vi "write_parameteres_to_file.vi"(0 "error 2":errorcluster, 8 "error":errorcluster, 11 "vi path":path) -> ()   [LabVIEW 2019]
panel:
  in  "data values 3":variant[](array[variant])
  in  "data values 2":variant[](array[variant])
  out "save path":string
  in  "data values":variant[](array[variant])
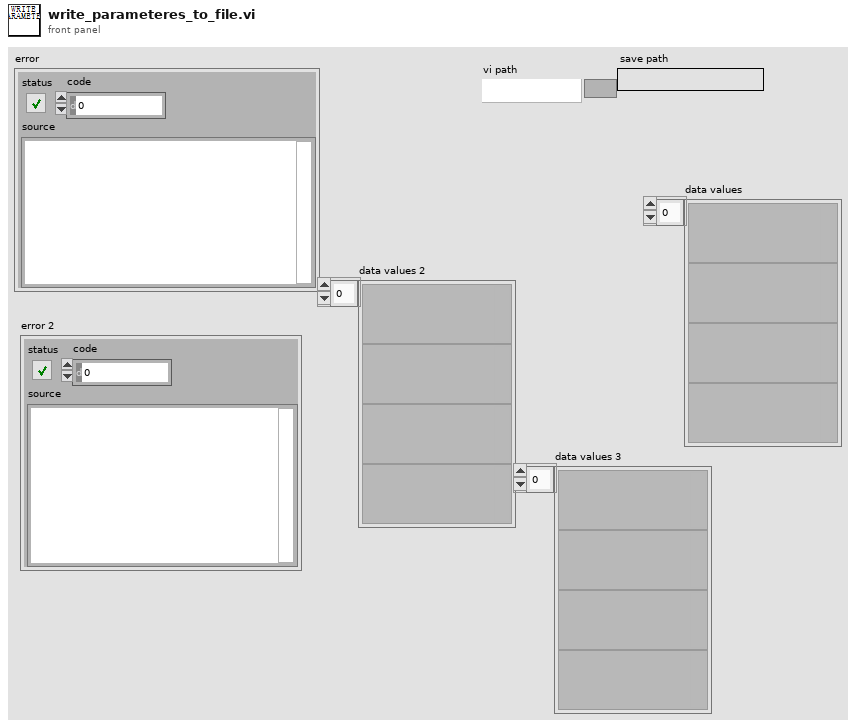
[diagram p1: front panel]
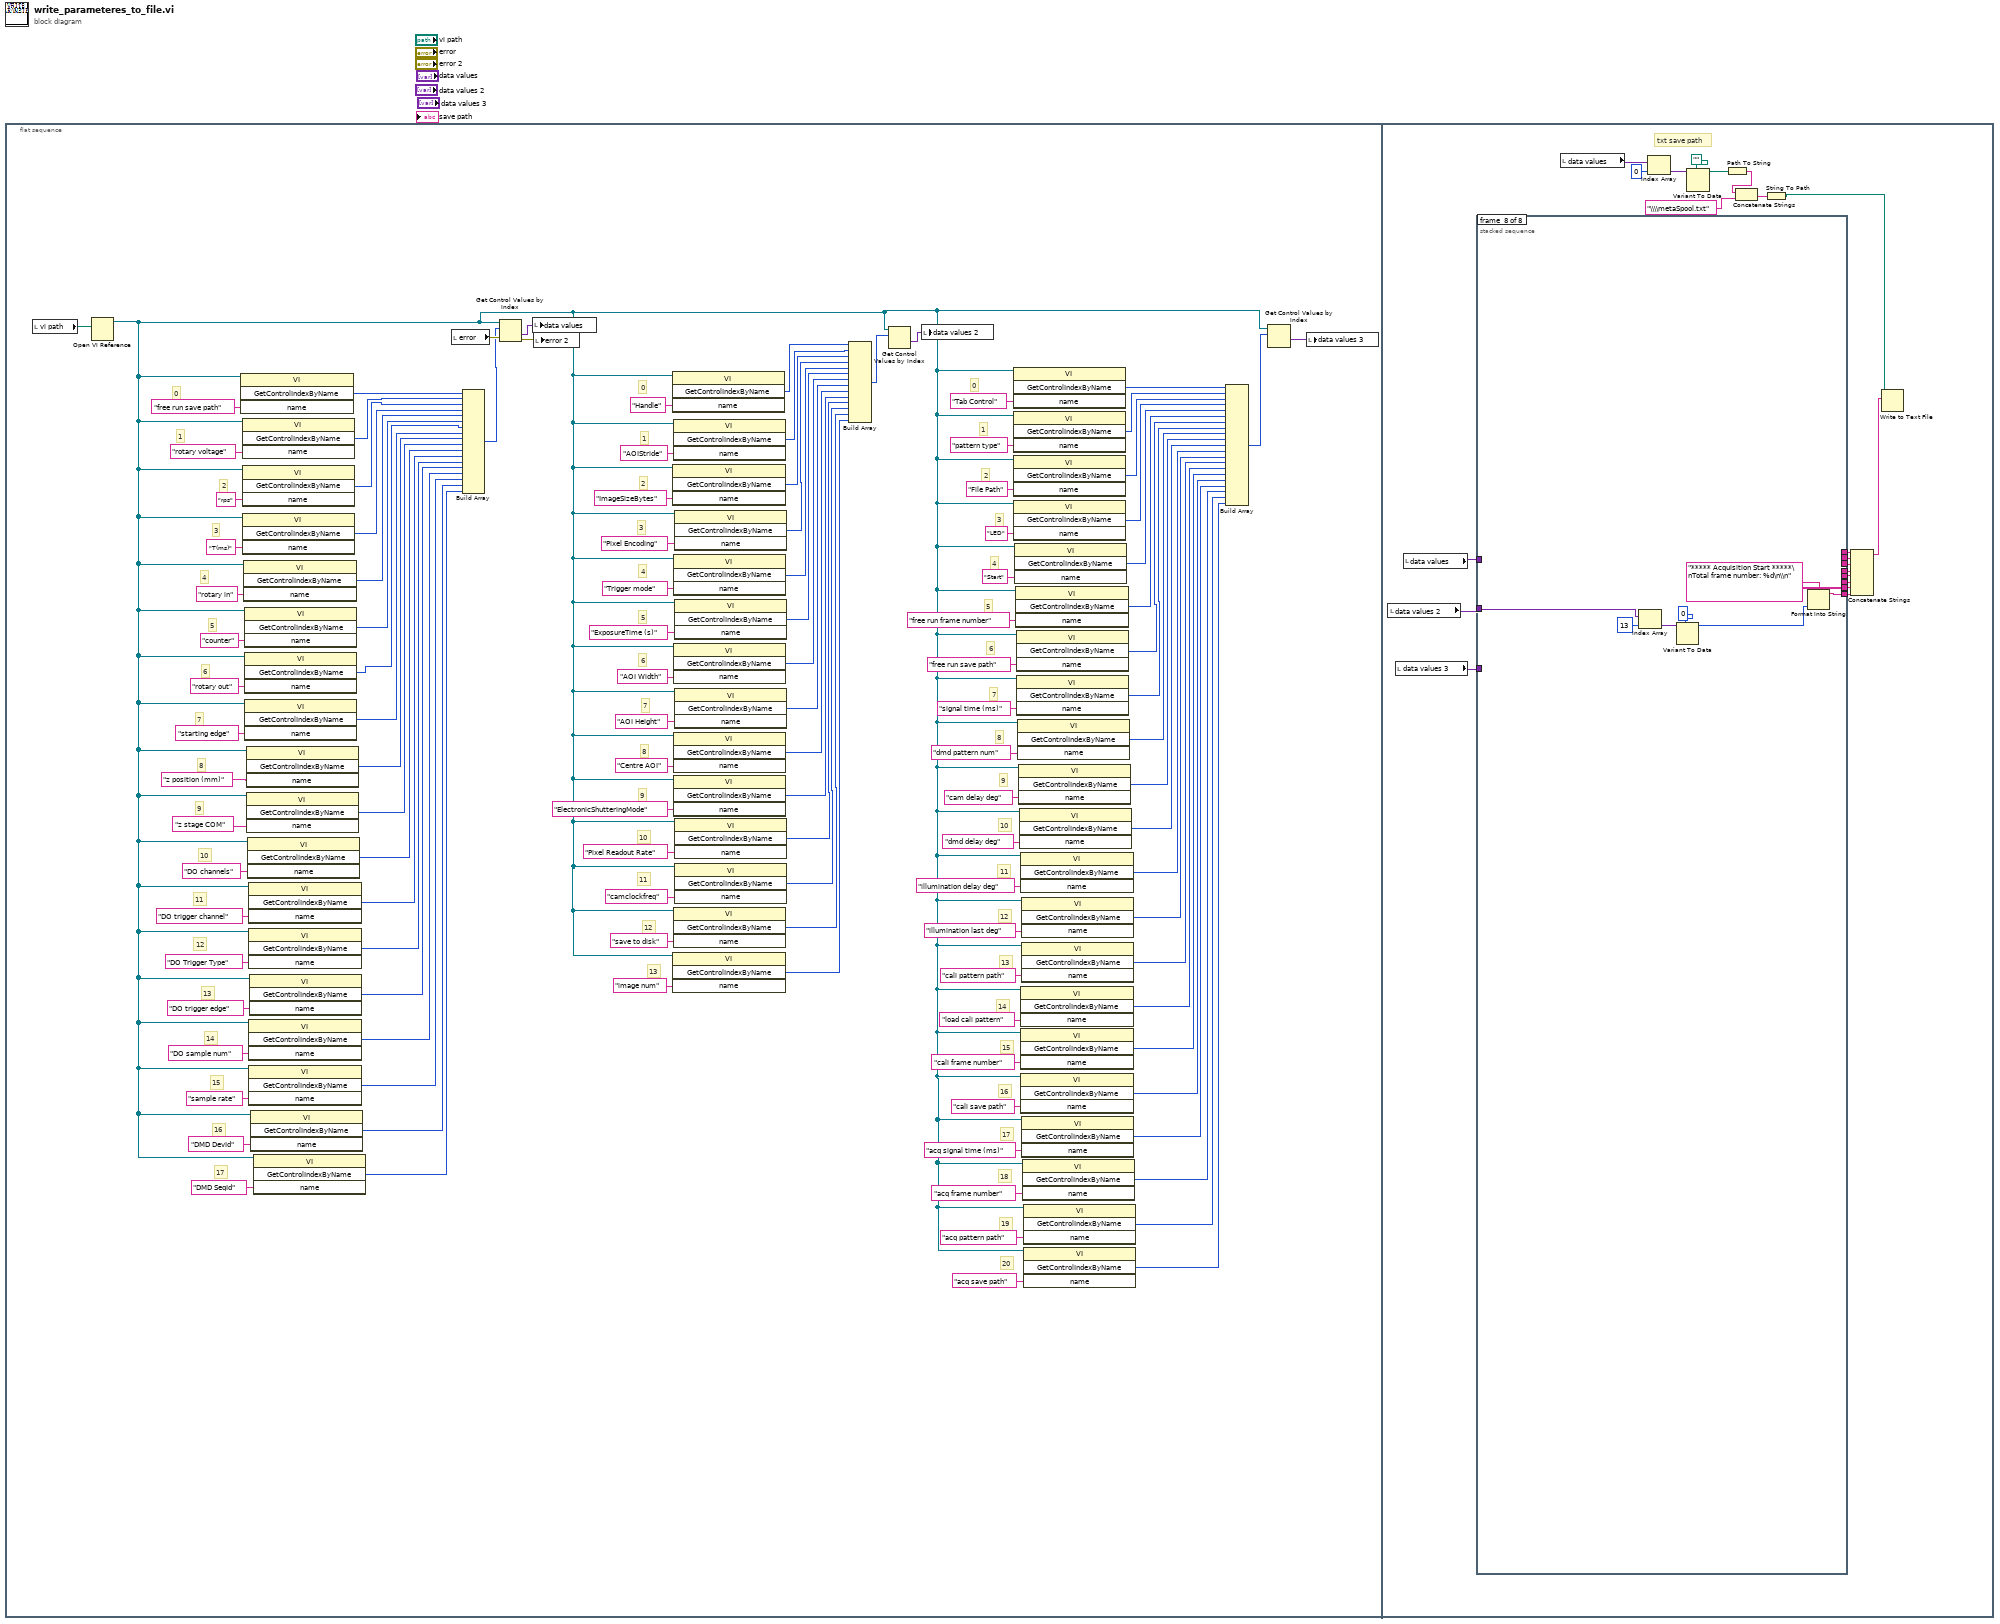
[diagram p0: block diagram]
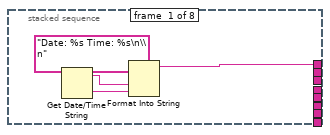
[diagram p2: hidden frame]
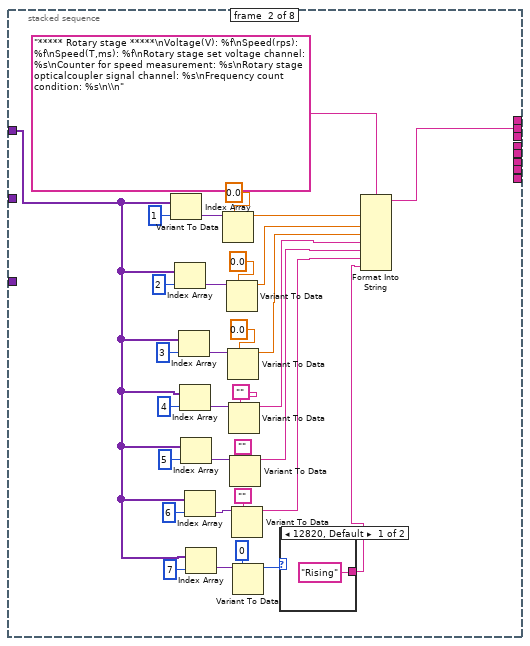
[diagram p3: hidden frame]
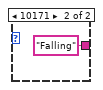
[diagram p4: hidden frame]
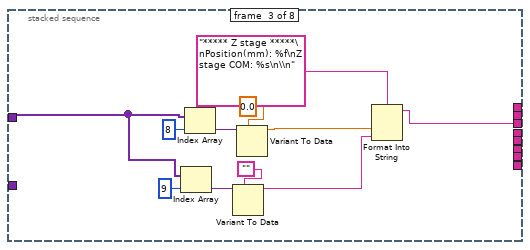
[diagram p5: hidden frame]
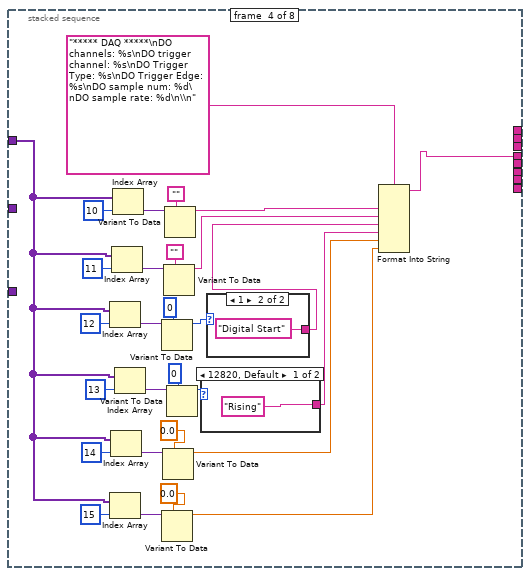
[diagram p6: hidden frame]
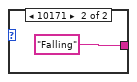
[diagram p7: hidden frame]
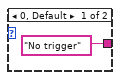
[diagram p8: hidden frame]
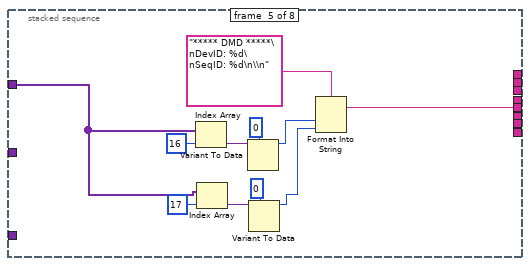
[diagram p9: hidden frame]
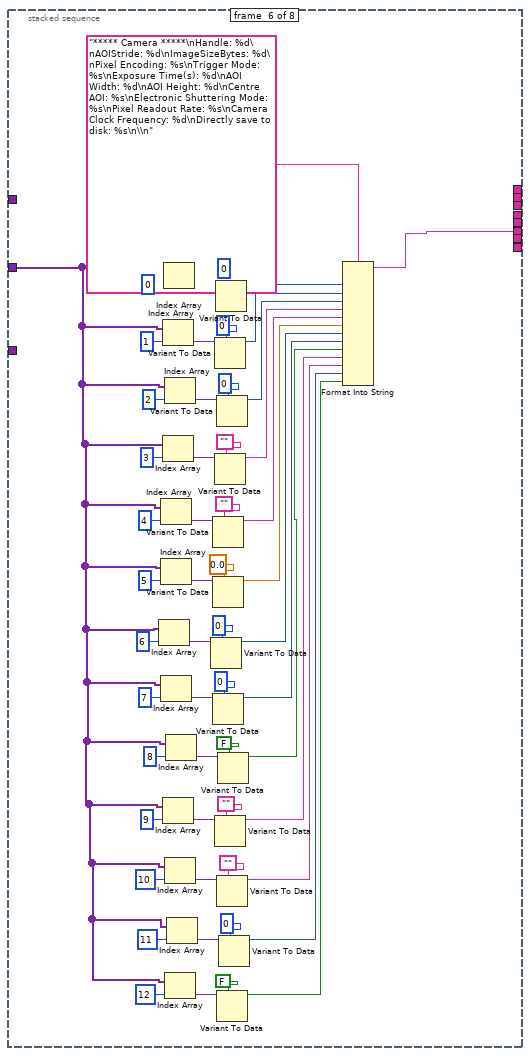
[diagram p10: hidden frame]
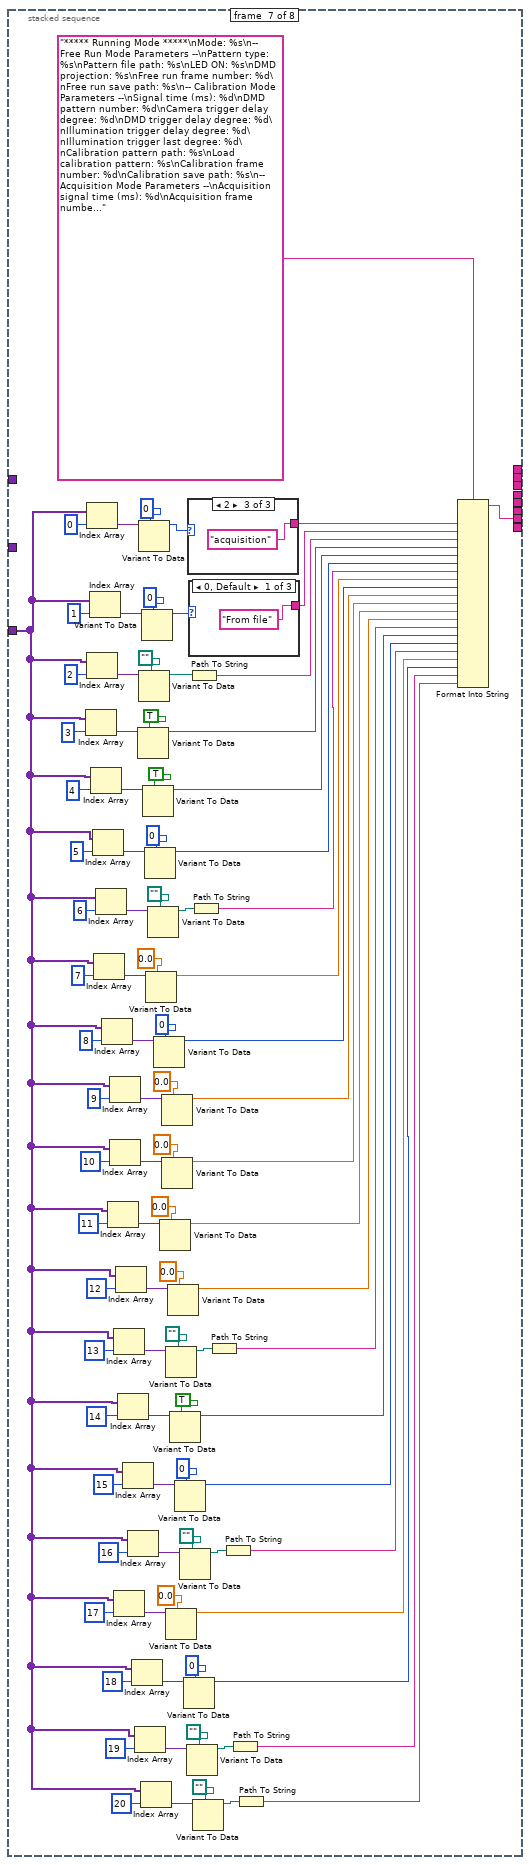
[diagram p11: hidden frame]
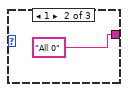
[diagram p12: hidden frame]
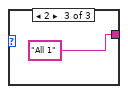
[diagram p13: hidden frame]
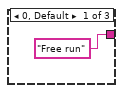
[diagram p14: hidden frame]
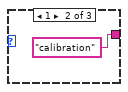
[diagram p15: hidden frame]
diagram:
  n1 = flat-sequence {
    frame #0 {
      # "13"
      # "15"
      # "20"
      # "19"
      # "18"
      # "17"
      # "16"
      # "14"
      # "13"
      # "12"
      # "11"
      # "10"
      # "9"
      # "8"
      # "7"
      # "6"
      # "5"
      # "4"
      # "3"
      # "2"
      # "1"
      # "12"
      # "0"
      # "11"
      # "10"
      # "9"
      # "8"
      # "7"
      # "6"
      # "5"
      # "4"
      # "3"
      # "2"
      # "1"
      # "0"
      # "17"
      # "16"
      # "15"
      # "14"
      # "13"
      # "12"
      # "11"
      # "10"
      # "9"
      # "8"
      # "7"
      # "6"
      # "5"
      # "4"
      # "3"
      # "2"
      # "1"
      # "0"
      n2 = local read "vi path"() -> (w116:path)
      n3 = Open VI Reference(vi path=w116) -> (vi reference=w2:refnum<vi>)  [unwired: 5 in, 1 out]
      n4 = invoke class="VI" method="GetControlIndexByName"(reference=w2, "name"="free run save path" ("Control Name")) -> ("GetControlIndexByName"=w108:i32)  [unwired: 2 in, 3 out]
      n5 = invoke class="VI" method="GetControlIndexByName"(reference=w2, "name"="rotary voltage" ("Control Name")) -> ("GetControlIndexByName"=w110:i32)  [unwired: 2 in, 3 out]
      n6 = invoke class="VI" method="GetControlIndexByName"(reference=w2, "name"="rps" ("Control Name")) -> ("GetControlIndexByName"=w105:i32)  [unwired: 2 in, 3 out]
      n7 = invoke class="VI" method="GetControlIndexByName"(reference=w2, "name"="T(ms)" ("Control Name")) -> ("GetControlIndexByName"=w104:i32)  [unwired: 2 in, 3 out]
      n8 = invoke class="VI" method="GetControlIndexByName"(reference=w2, "name"="rotary in" ("Control Name")) -> ("GetControlIndexByName"=w102:i32)  [unwired: 2 in, 3 out]
      n9 = invoke class="VI" method="GetControlIndexByName"(reference=w2, "name"="counter" ("Control Name")) -> ("GetControlIndexByName"=w100:i32)  [unwired: 2 in, 3 out]
      n10 = invoke class="VI" method="GetControlIndexByName"(reference=w2, "name"="rotary out" ("Control Name")) -> ("GetControlIndexByName"=w98:i32)  [unwired: 2 in, 3 out]
      n11 = invoke class="VI" method="GetControlIndexByName"(reference=w2, "name"="starting edge" ("Control Name")) -> ("GetControlIndexByName"=w97:i32)  [unwired: 2 in, 3 out]
      n12 = invoke class="VI" method="GetControlIndexByName"(reference=w2, "name"="z position (mm)" ("Control Name")) -> ("GetControlIndexByName"=w95:i32)  [unwired: 2 in, 3 out]
      n13 = invoke class="VI" method="GetControlIndexByName"(reference=w2, "name"="z stage COM" ("Control Name")) -> ("GetControlIndexByName"=w94:i32)  [unwired: 2 in, 3 out]
      n14 = invoke class="VI" method="GetControlIndexByName"(reference=w2, "name"="DO channels" ("Control Name")) -> ("GetControlIndexByName"=w83:i32)  [unwired: 2 in, 3 out]
      n15 = invoke class="VI" method="GetControlIndexByName"(reference=w2, "name"="DO trigger channel" ("Control Name")) -> ("GetControlIndexByName"=w82:i32)  [unwired: 2 in, 3 out]
      n16 = invoke class="VI" method="GetControlIndexByName"(reference=w2, "name"="DO Trigger Type" ("Control Name")) -> ("GetControlIndexByName"=w81:i32)  [unwired: 2 in, 3 out]
      n17 = invoke class="VI" method="GetControlIndexByName"(reference=w2, "name"="DO sample num" ("Control Name")) -> ("GetControlIndexByName"=w79:i32)  [unwired: 2 in, 3 out]
      n18 = invoke class="VI" method="GetControlIndexByName"(reference=w2, "name"="sample rate" ("Control Name")) -> ("GetControlIndexByName"=w78:i32)  [unwired: 2 in, 3 out]
      n19 = invoke class="VI" method="GetControlIndexByName"(reference=w2, "name"="DO trigger edge" ("Control Name")) -> ("GetControlIndexByName"=w80:i32)  [unwired: 2 in, 3 out]
      n20 = invoke class="VI" method="GetControlIndexByName"(reference=w2, "name"="DMD DevId" ("Control Name")) -> ("GetControlIndexByName"=w77:i32)  [unwired: 2 in, 3 out]
      n21 = invoke class="VI" method="GetControlIndexByName"(reference=w2, "name"="DMD SeqId" ("Control Name")) -> ("GetControlIndexByName"=w76:i32)  [unwired: 2 in, 3 out]
      n22 = local read "error"() -> (w115:errorcluster)
      n23 = Build Array(w108, w110, w105, w104, w102, w100, w98, w97, w95, w94, w83, w82, w81, w80, w79, w78, w77, w76) -> (w112:i32[])
      n24 = Get Control Values by Index(0:w2, 1:w112, 3:w115) -> (10:w109:variant[], 11:w114:errorcluster)
      n25 = local write "data values"(w109) -> ()
      n26 = local write "error 2"(w114) -> ()
      n27 = invoke class="VI" method="GetControlIndexByName"(reference=w2, "name"="Handle" ("Control Name")) -> ("GetControlIndexByName"=w73:i32)  [unwired: 2 in, 3 out]
      n28 = invoke class="VI" method="GetControlIndexByName"(reference=w2, "name"="ImageSizeBytes" ("Control Name")) -> ("GetControlIndexByName"=w59:i32)  [unwired: 2 in, 3 out]
      n29 = invoke class="VI" method="GetControlIndexByName"(reference=w2, "name"="image num" ("Control Name")) -> ("GetControlIndexByName"=w1:i32)  [unwired: 2 in, 3 out]
      n30 = invoke class="VI" method="GetControlIndexByName"(reference=w2, "name"="AOIStride" ("Control Name")) -> ("GetControlIndexByName"=w70:i32)  [unwired: 2 in, 3 out]
      n31 = invoke class="VI" method="GetControlIndexByName"(reference=w2, "name"="Trigger mode" ("Control Name")) -> ("GetControlIndexByName"=w57:i32)  [unwired: 2 in, 3 out]
      n32 = invoke class="VI" method="GetControlIndexByName"(reference=w2, "name"="AOI Width" ("Control Name")) -> ("GetControlIndexByName"=w55:i32)  [unwired: 2 in, 3 out]
      n33 = invoke class="VI" method="GetControlIndexByName"(reference=w2, "name"="Centre AOI" ("Control Name")) -> ("GetControlIndexByName"=w53:i32)  [unwired: 2 in, 3 out]
      n34 = invoke class="VI" method="GetControlIndexByName"(reference=w2, "name"="ElectronicShutteringMode" ("Control Name")) -> ("GetControlIndexByName"=w52:i32)  [unwired: 2 in, 3 out]
      n35 = invoke class="VI" method="GetControlIndexByName"(reference=w2, "name"="save to disk" ("Control Name")) -> ("GetControlIndexByName"=w38:i32)  [unwired: 2 in, 3 out]
      n36 = invoke class="VI" method="GetControlIndexByName"(reference=w2, "name"="Pixel Encoding" ("Control Name")) -> ("GetControlIndexByName"=w58:i32)  [unwired: 2 in, 3 out]
      n37 = invoke class="VI" method="GetControlIndexByName"(reference=w2, "name"="ExposureTime (s)" ("Control Name")) -> ("GetControlIndexByName"=w56:i32)  [unwired: 2 in, 3 out]
      n38 = invoke class="VI" method="GetControlIndexByName"(reference=w2, "name"="AOI Height" ("Control Name")) -> ("GetControlIndexByName"=w54:i32)  [unwired: 2 in, 3 out]
      n39 = invoke class="VI" method="GetControlIndexByName"(reference=w2, "name"="Pixel Readout Rate" ("Control Name")) -> ("GetControlIndexByName"=w51:i32)  [unwired: 2 in, 3 out]
      n40 = invoke class="VI" method="GetControlIndexByName"(reference=w2, "name"="camclockfreq" ("Control Name")) -> ("GetControlIndexByName"=w50:i32)  [unwired: 2 in, 3 out]
      n41 = Build Array(w73, w70, w59, w58, w57, w56, w55, w54, w53, w52, w51, w50, w38, w1) -> (w74:i32[])
      n42 = Get Control Values by Index(0:w2, 1:w74) -> (10:w75:variant[])  [unwired: 1 in, 1 out]
      n43 = local write "data values 2"(w75) -> ()
      n44 = invoke class="VI" method="GetControlIndexByName"(reference=w2, "name"="Tab Control" ("Control Name")) -> ("GetControlIndexByName"=w48:i32)  [unwired: 2 in, 3 out]
      n45 = invoke class="VI" method="GetControlIndexByName"(reference=w2, "name"="pattern type" ("Control Name")) -> ("GetControlIndexByName"=w33:i32)  [unwired: 2 in, 3 out]
      n46 = invoke class="VI" method="GetControlIndexByName"(reference=w2, "name"="File Path" ("Control Name")) -> ("GetControlIndexByName"=w32:i32)  [unwired: 2 in, 3 out]
      n47 = invoke class="VI" method="GetControlIndexByName"(reference=w2, "name"="LED" ("Control Name")) -> ("GetControlIndexByName"=w31:i32)  [unwired: 2 in, 3 out]
      n48 = invoke class="VI" method="GetControlIndexByName"(reference=w2, "name"="Start" ("Control Name")) -> ("GetControlIndexByName"=w30:i32)  [unwired: 2 in, 3 out]
      n49 = invoke class="VI" method="GetControlIndexByName"(reference=w2, "name"="free run frame number" ("Control Name")) -> ("GetControlIndexByName"=w29:i32)  [unwired: 2 in, 3 out]
      n50 = invoke class="VI" method="GetControlIndexByName"(reference=w2, "name"="free run save path" ("Control Name")) -> ("GetControlIndexByName"=w28:i32)  [unwired: 2 in, 3 out]
      n51 = invoke class="VI" method="GetControlIndexByName"(reference=w2, "name"="signal time (ms)" ("Control Name")) -> ("GetControlIndexByName"=w27:i32)  [unwired: 2 in, 3 out]
      n52 = invoke class="VI" method="GetControlIndexByName"(reference=w2, "name"="dmd pattern num" ("Control Name")) -> ("GetControlIndexByName"=w26:i32)  [unwired: 2 in, 3 out]
      n53 = invoke class="VI" method="GetControlIndexByName"(reference=w2, "name"="cam delay deg" ("Control Name")) -> ("GetControlIndexByName"=w25:i32)  [unwired: 2 in, 3 out]
      n54 = invoke class="VI" method="GetControlIndexByName"(reference=w2, "name"="dmd delay deg" ("Control Name")) -> ("GetControlIndexByName"=w24:i32)  [unwired: 2 in, 3 out]
      n55 = invoke class="VI" method="GetControlIndexByName"(reference=w2, "name"="illumination delay deg" ("Control Name")) -> ("GetControlIndexByName"=w18:i32)  [unwired: 2 in, 3 out]
      n56 = invoke class="VI" method="GetControlIndexByName"(reference=w2, "name"="load cali pattern" ("Control Name")) -> ("GetControlIndexByName"=w15:i32)  [unwired: 2 in, 3 out]
      n57 = invoke class="VI" method="GetControlIndexByName"(reference=w2, "name"="cali frame number" ("Control Name")) -> ("GetControlIndexByName"=w6:i32)  [unwired: 2 in, 3 out]
      n58 = invoke class="VI" method="GetControlIndexByName"(reference=w2, "name"="cali save path" ("Control Name")) -> ("GetControlIndexByName"=w5:i32)  [unwired: 2 in, 3 out]
      n59 = invoke class="VI" method="GetControlIndexByName"(reference=w2, "name"="illumination last deg" ("Control Name")) -> ("GetControlIndexByName"=w17:i32)  [unwired: 2 in, 3 out]
      n60 = invoke class="VI" method="GetControlIndexByName"(reference=w2, "name"="cali pattern path" ("Control Name")) -> ("GetControlIndexByName"=w16:i32)  [unwired: 2 in, 3 out]
      n61 = invoke class="VI" method="GetControlIndexByName"(reference=w2, "name"="acq signal time (ms)" ("Control Name")) -> ("GetControlIndexByName"=w4:i32)  [unwired: 2 in, 3 out]
      n62 = invoke class="VI" method="GetControlIndexByName"(reference=w2, "name"="acq frame number" ("Control Name")) -> ("GetControlIndexByName"=w7:i32)  [unwired: 2 in, 3 out]
      n63 = invoke class="VI" method="GetControlIndexByName"(reference=w2, "name"="acq pattern path" ("Control Name")) -> ("GetControlIndexByName"=w8:i32)  [unwired: 2 in, 3 out]
      n64 = invoke class="VI" method="GetControlIndexByName"(reference=w2, "name"="acq save path" ("Control Name")) -> ("GetControlIndexByName"=w9:i32)  [unwired: 2 in, 3 out]
      n65 = Build Array(w48, w33, w32, w31, w30, w29, w28, w27, w26, w25, w24, w18, w17, w16, w15, w6, w5, w4, w7, w8, w9) -> (w47:i32[])
      n66 = Get Control Values by Index(0:w2, 1:w47) -> (10:w49:variant[])  [unwired: 1 in, 1 out]
      n67 = local write "data values 3"(w49) -> ()
    }
    frame #1 {
      # "txt save path"
      n68 = local read "data values 2"() -> (w120:variant[])
      n69 = local read "data values 3"() -> (w118:variant[])
      n70 = local read "data values"() -> (w124:variant[])
      n71 = stacked-sequence {
        tunnel: [w138 _ _ _ _ _ _ _] -> w127
        tunnel: [_ w143 _ _ _ _ _ _] -> w126
        tunnel: [_ _ w177 _ _ _ _ _] -> w125
        tunnel: w124 -> [_ w142 w176 w188 w220 _ _ _]
        tunnel: [_ _ _ w204 _ _ _ _] -> w123
        tunnel: [_ _ _ _ w230 _ _ _] -> w122
        tunnel: [_ _ _ _ _ w281 _ _] -> w121
        tunnel: w120 -> [_ _ _ _ _ w232 _ w387]
        tunnel: [_ _ _ _ _ _ w377 _] -> w119
        tunnel: w118 -> [_ _ _ _ _ _ w296 _]
        tunnel: [_ _ _ _ _ _ _ w393] -> w117
        frame #0 {
          n72 = Get Date/Time String() -> (date string=w140:string, time string=w141:string)  [unwired: 3 in]
          n73 = Format Into String(format string="Date: %s Time: %s\n\\n", w140, w141) -> (resulting string=w138:string)  [unwired: 2 in, 1 out]
        }
        frame #1 {
          n74 = Index Array(array=w142, index=1) -> (element=w159:variant)
          n75 = Index Array(array=w142, index=2) -> (element=w161:variant)
          n76 = Index Array(array=w142, index=3) -> (element=w163:variant)
          n77 = Index Array(array=w142, index=4) -> (element=w165:variant)
          n78 = Index Array(array=w142, index=5) -> (element=w167:variant)
          n79 = Index Array(array=w142, index=6) -> (element=w169:variant)
          n80 = Index Array(array=w142, index=7) -> (element=w170:variant)
          n81 = Variant To Data(type=0.0, Variant=w159) -> (data=w160:dbl)  [unwired: 1 in, 1 out]
          n82 = Variant To Data(type=0.0, Variant=w161) -> (data=w162:dbl)  [unwired: 1 in, 1 out]
          n83 = Variant To Data(type=0.0, Variant=w163) -> (data=w164:dbl)  [unwired: 1 in, 1 out]
          n84 = Variant To Data(type="", Variant=w165) -> (data=w166:string)  [unwired: 1 in, 1 out]
          n85 = Variant To Data(type="", Variant=w167) -> (data=w168:string)  [unwired: 1 in, 1 out]
          n86 = Variant To Data(type="", Variant=w169) -> (data=w171:string)  [unwired: 1 in, 1 out]
          n87 = Variant To Data(type=0, Variant=w170) -> (data=w172:i32)  [unwired: 1 in, 1 out]
          n88 = case shown="12820, Default" w172 {
            tunnel: ["Rising" "Falling"] -> w173
            frame 12820, Default {
            }
            frame 10171 {
            }
          }
          n89 = Format Into String(format string="***** Rotary stage *****\nVoltage(V): %f\nSpeed(rps): %f\nSpeed(T,ms): %f\nRotary stage set voltage channel: %s\nCounter for speed measurement: %s\nRotary stage opticalcoupler signal channel: %s\nFrequency count condition: %s\n\\n", w160, w162, w164, w166, w168, w171, w173) -> (resulting string=w143:string)  [unwired: 2 in, 1 out]
        }
        frame #2 {
          n90 = Index Array(array=w176, index=9) -> (element=w185:variant)
          n91 = Index Array(array=w176, index=8) -> (element=w183:variant)
          n92 = Variant To Data(type="", Variant=w185) -> (data=w186:string)  [unwired: 1 in, 1 out]
          n93 = Variant To Data(type=0.0, Variant=w183) -> (data=w184:dbl)  [unwired: 1 in, 1 out]
          n94 = Format Into String(format string="***** Z stage *****\nPosition(mm): %f\nZ stage COM: %s\n\\n", w184, w186) -> (resulting string=w177:string)  [unwired: 2 in, 1 out]
        }
        frame #3 {
          n95 = Index Array(array=w188, index=12) -> (element=w207:variant)
          n96 = Index Array(array=w188, index=15) -> (element=w192:variant)
          n97 = Index Array(array=w188, index=14) -> (element=w195:variant)
          n98 = Index Array(array=w188, index=11) -> (element=w210:variant)
          n99 = Index Array(array=w188, index=10) -> (element=w215:variant)
          n100 = Index Array(array=w188, index=13) -> (element=w200:variant)
          n101 = Variant To Data(type=0, Variant=w207) -> (data=w202:i32)  [unwired: 1 in, 1 out]
          n102 = Variant To Data(type=0.0, Variant=w192) -> (data=w187:dbl)  [unwired: 1 in, 1 out]
          n103 = Variant To Data(type=0.0, Variant=w195) -> (data=w193:dbl)  [unwired: 1 in, 1 out]
          n104 = Variant To Data(type="", Variant=w210) -> (data=w205:string)  [unwired: 1 in, 1 out]
          n105 = Variant To Data(type="", Variant=w215) -> (data=w211:string)  [unwired: 1 in, 1 out]
          n106 = Variant To Data(type=0, Variant=w200) -> (data=w197:i32)  [unwired: 1 in, 1 out]
          n107 = case shown="12820, Default" w197 {
            tunnel: ["Rising" "Falling"] -> w196
            frame 12820, Default {
            }
            frame 10171 {
            }
          }
          n108 = case shown="1" w202 {
            tunnel: ["No trigger" "Digital Start"] -> w201
            frame 0, Default {
            }
            frame 1 {
            }
          }
          n109 = Format Into String(format string="***** DAQ *****\nDO channels: %s\nDO trigger channel: %s\nDO Trigger Type: %s\nDO Trigger Edge: %s\nDO sample num: %d\nDO sample rate: %d\n\\n", w211, w205, w201, w196, w193, w187) -> (resulting string=w204:string)  [unwired: 2 in, 1 out]
        }
        frame #4 {
          n110 = Index Array(array=w220, index=16) -> (element=w228:variant)
          n111 = Index Array(array=w220, index=17) -> (element=w224:variant)
          n112 = Variant To Data(type=0, Variant=w228) -> (data=w225:i32)  [unwired: 1 in, 1 out]
          n113 = Variant To Data(type=0, Variant=w224) -> (data=w221:i32)  [unwired: 1 in, 1 out]
          n114 = Format Into String(format string="***** DMD *****\nDevID: %d\nSeqID: %d\n\\n", w225, w221) -> (resulting string=w230:string)  [unwired: 2 in, 1 out]
        }
        frame #5 {
          n115 = Index Array(array=w232, index=6) -> (element=w267:variant)
          n116 = Index Array(array=w232, index=4) -> (element=w271:variant)
          n117 = Index Array(array=w232, index=5) -> (element=w269:variant)
          n118 = Index Array(array=w232, index=7) -> (element=w255:variant)
          n119 = Index Array(array=w232, index=1) -> (element=w279:variant)
          n120 = Index Array(array=w232, index=3) -> (element=w273:variant)
          n121 = Index Array(array=w232, index=9) -> (element=w250:variant)
          n122 = Index Array(array=w232, index=0) -> (element=w285:variant)
          n123 = Index Array(array=w232, index=2) -> (element=w276:variant)
          n124 = Index Array(array=w232, index=10) -> (element=w248:variant)
          n125 = Index Array(array=w232, index=12) -> (element=w235:variant)
          n126 = Index Array(array=w232, index=8) -> (element=w252:variant)
          n127 = Index Array(array=w232, index=11) -> (element=w246:variant)
          n128 = Variant To Data(type=0, Variant=w267) -> (data=w256:i32)  [unwired: 1 in, 1 out]
          n129 = Variant To Data(type="", Variant=w271) -> (data=w259:string)  [unwired: 1 in, 1 out]
          n130 = Variant To Data(type=0.0, Variant=w269) -> (data=w257:dbl)  [unwired: 1 in, 1 out]
          n131 = Variant To Data(type=0, Variant=w255) -> (data=w243:i32)  [unwired: 1 in, 1 out]
          n132 = Variant To Data(type=0, Variant=w279) -> (data=w264:i32)  [unwired: 1 in, 1 out]
          n133 = Variant To Data(type="", Variant=w273) -> (data=w261:string)  [unwired: 1 in, 1 out]
          n134 = Variant To Data(type="", Variant=w250) -> (data=w241:string)  [unwired: 1 in, 1 out]
          n135 = Variant To Data(type=0, Variant=w285) -> (data=w282:i32)  [unwired: 1 in, 1 out]
          n136 = Variant To Data(type=0, Variant=w276) -> (data=w263:i32)  [unwired: 1 in, 1 out]
          n137 = Variant To Data(type="", Variant=w248) -> (data=w238:string)  [unwired: 1 in, 1 out]
          n138 = Variant To Data(type=FALSE, Variant=w235) -> (data=w231:bool)  [unwired: 1 in, 1 out]
          n139 = Variant To Data(type=FALSE, Variant=w252) -> (data=w242:bool)  [unwired: 1 in, 1 out]
          n140 = Variant To Data(type=0, Variant=w246) -> (data=w237:i32)  [unwired: 1 in, 1 out]
          n141 = Format Into String(format string="***** Camera *****\nHandle: %d\nAOIStride: %d\nImageSizeBytes: %d\nPixel Encoding: %s\nTrigger Mode: %s\nExposure Time(s): %d\nAOI Width: %d\nAOI Height: %d\nCentre AOI: %s\nElectronic Shuttering Mode: %s\nPixel Readout Rate: %s\nCamera Clock Frequency: %d\nDirectly save to disk: %s\n\\n", w282, w264, w263, w261, w259, w257, w256, w243, w242, w241, w238, w237, w231) -> (resulting string=w281:string)  [unwired: 2 in, 1 out]
        }
        frame #6 {
          n142 = Index Array(array=w296, index=3) -> (element=w368:variant)
          n143 = Index Array(array=w296, index=0) -> (element=w380:variant)
          n144 = Index Array(array=w296, index=2) -> (element=w365:variant)
          n145 = Index Array(array=w296, index=1) -> (element=w373:variant)
          n146 = Index Array(array=w296, index=4) -> (element=w359:variant)
          n147 = Index Array(array=w296, index=5) -> (element=w355:variant)
          n148 = Index Array(array=w296, index=7) -> (element=w346:variant)
          n149 = Index Array(array=w296, index=6) -> (element=w352:variant)
          n150 = Index Array(array=w296, index=8) -> (element=w343:variant)
          n151 = Index Array(array=w296, index=11) -> (element=w334:variant)
          n152 = Index Array(array=w296, index=9) -> (element=w340:variant)
          n153 = Index Array(array=w296, index=10) -> (element=w337:variant)
          n154 = Index Array(array=w296, index=13) -> (element=w324:variant)
          n155 = Index Array(array=w296, index=17) -> (element=w310:variant)
          n156 = Index Array(array=w296, index=12) -> (element=w327:variant)
          n157 = Index Array(array=w296, index=14) -> (element=w320:variant)
          n158 = Index Array(array=w296, index=15) -> (element=w317:variant)
          n159 = Index Array(array=w296, index=16) -> (element=w314:variant)
          n160 = Index Array(array=w296, index=18) -> (element=w307:variant)
          n161 = Index Array(array=w296, index=19) -> (element=w304:variant)
          n162 = Variant To Data(type=TRUE, Variant=w368) -> (data=w360:bool)  [unwired: 1 in, 1 out]
          n163 = Variant To Data(type=0, Variant=w380) -> (data=w375:i32)  [unwired: 1 in, 1 out]
          n164 = Variant To Data(type=path "", Variant=w365) -> (data=w362:path)  [unwired: 1 in, 1 out]
          n165 = Index Array(array=w296, index=20) -> (element=w300:variant)
          n166 = Variant To Data(type=0, Variant=w373) -> (data=w371:i32)  [unwired: 1 in, 1 out]
          n167 = Variant To Data(type=TRUE, Variant=w359) -> (data=w357:bool)  [unwired: 1 in, 1 out]
          n168 = Variant To Data(type=0, Variant=w355) -> (data=w348:i32)  [unwired: 1 in, 1 out]
          n169 = Variant To Data(type=0.0, Variant=w346) -> (data=w331:dbl)  [unwired: 1 in, 1 out]
          n170 = Variant To Data(type=path "", Variant=w352) -> (data=w349:path)  [unwired: 1 in, 1 out]
          n171 = Variant To Data(type=0, Variant=w343) -> (data=w330:i32)  [unwired: 1 in, 1 out]
          n172 = Variant To Data(type=0.0, Variant=w334) -> (data=w295:dbl)  [unwired: 1 in, 1 out]
          n173 = Variant To Data(type=0.0, Variant=w340) -> (data=w329:dbl)  [unwired: 1 in, 1 out]
          n174 = Variant To Data(type=0.0, Variant=w337) -> (data=w328:dbl)  [unwired: 1 in, 1 out]
          n175 = Variant To Data(type=path "", Variant=w324) -> (data=w321:path)  [unwired: 1 in, 1 out]
          n176 = Variant To Data(type=0.0, Variant=w310) -> (data=w289:dbl)  [unwired: 1 in, 1 out]
          n177 = Variant To Data(type=0.0, Variant=w327) -> (data=w294:dbl)  [unwired: 1 in, 1 out]
          n178 = Variant To Data(type=TRUE, Variant=w320) -> (data=w292:bool)  [unwired: 1 in, 1 out]
          n179 = Variant To Data(type=0, Variant=w317) -> (data=w291:i32)  [unwired: 1 in, 1 out]
          n180 = Variant To Data(type=path "", Variant=w314) -> (data=w311:path)  [unwired: 1 in, 1 out]
          n181 = Variant To Data(type=0, Variant=w307) -> (data=w288:i32)  [unwired: 1 in, 1 out]
          n182 = Variant To Data(type=path "", Variant=w304) -> (data=w301:path)  [unwired: 1 in, 1 out]
          n183 = case shown="2" w375 {
            tunnel: ["Free run" "calibration" "acquisition"] -> w374
            frame 0, Default {
            }
            frame 1 {
            }
            frame 2 {
            }
          }
          n184 = case shown="0, Default" w371 {
            tunnel: ["From file" "All 0" "All 1"] -> w370
            frame 0, Default {
            }
            frame 1 {
            }
            frame 2 {
            }
          }
          n185 = Path To String(path=w362) -> (string=w361:string)
          n186 = Path To String(path=w349) -> (string=w347:string)
          n187 = Variant To Data(type=path "", Variant=w300) -> (data=w297:path)  [unwired: 1 in, 1 out]
          n188 = Path To String(path=w321) -> (string=w293:string)
          n189 = Path To String(path=w311) -> (string=w290:string)
          n190 = Path To String(path=w301) -> (string=w287:string)
          n191 = Path To String(path=w297) -> (string=w286:string)
          n192 = Format Into String(format string="***** Running Mode *****\nMode: %s\n-- Free Run Mode Parameters --\nPattern type: %s\nPattern file path: %s\nLED ON: %s\nDMD projection: %s\nFree run frame number: %d\nFree run save path: %s\n-- Calibration Mode Parameters --\nSignal time (ms): %d\nDMD pattern number: %d\nCamera trigger delay degree: %d\nDMD trigger delay degree: %d\nIllumination trigger delay degree: %d\nIllumination trigger last degree: %d\nCalibration pattern path: %s\nLoad calibration pattern: %s\nCalibration frame number: %d\nCalibration save path: %s\n-- Acquisition Mode Parameters --\nAcquisition signal time (ms): %d\nAcquisition frame number: %d\nAcquisition pattern path: %s\nAcquisition save path: %s\n\\n", w374, w370, w361, w360, w357, w348, w347, w331, w330, w329, w328, w295, w294, w293, w292, w291, w290, w289, w288, w287, w286) -> (resulting string=w377:string)  [unwired: 2 in, 1 out]
        }
        frame #7 {
          n193 = Index Array(array=w387, index=13) -> (element=w391:variant)
          n194 = Variant To Data(type=0, Variant=w391) -> (data=w388:i32)  [unwired: 1 in, 1 out]
          n195 = Format Into String(format string="***** Acquisition Start *****\nTotal frame number: %d\n\\n", w388) -> (resulting string=w393:string)  [unwired: 2 in, 1 out]
        }
      }
      n196 = local read "data values"() -> (w132:variant[])
      n197 = Index Array(array=w132, index=0) -> (element=w133:variant)
      n198 = Variant To Data(type=path "", Variant=w133) -> (data=w137:path)  [unwired: 1 in, 1 out]
      n199 = Path To String(path=w137) -> (string=w134:string)
      n200 = Concatenate Strings(w134, "\\\\metaSpool.txt" ("format string")) -> (w136:string)
      n201 = String To Path(string=w136) -> (path=w135:path)
      n202 = Concatenate Strings(w127, w126, w125, w123, w122, w121, w119, w117) -> (w128:string)
      n203 = Write to Text File(file (use dialog)=w135, text=w128) -> ()  [unwired: 2 in, 3 out]
    }
  }
